vi "MathematicaHandlerBindTest.vi"() -> ()   [LabVIEW 2014]
uses:
  <vilib>/event_ctls.llb/lveventtype.ctl
panel:
  out "Array":string[](array[string])
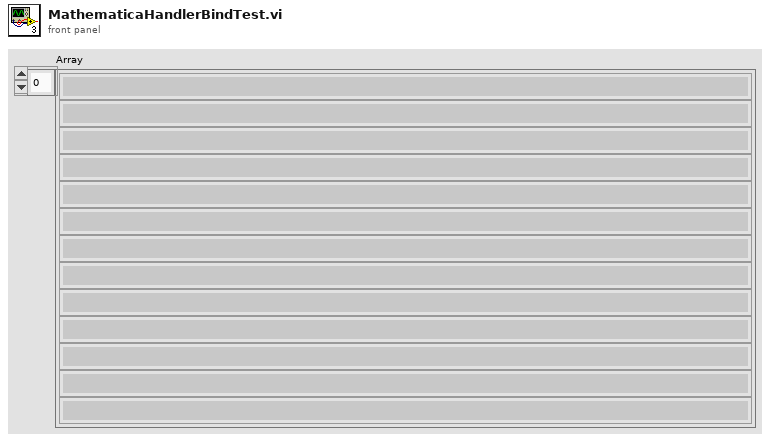
[diagram p1: front panel]
types:
  T1 = typedef "lveventtype.ctl" = enum32{"Null", "Timeout", "Annotation Menu Selection", "Annotation Menu Selection?", "App Instance Close", "App Instance Close?", "Autoscale Range Change", "Bookmark Info Change", "Cell Edit", "Cell Edit?", "Cursor Grab", "Cursor Grab?", "Cursor Menu Selection", "Cursor Menu Selection?", "Cursor Move", "Cursor Release", "Data Change", "Direction Change", "Display State Change", "Drag Ended", "Drag Enter", "Drag Leave", "Drag Over", "Drag Source Update", "Drag Starting", "Drag Starting?", "Drop", "Exec State Change", "Key Down", "Key Down?", "Key Repeat", "Key Repeat?", "Key Up", "Listbox Double Click", "Menu Activation?", "Menu Selection (App)", "Menu Selection? (App)", "Menu Selection (User)", "Mouse Down", "Mouse Down?", "Mouse Enter", "Mouse Leave", "Mouse Move", "Mouse Up", "Mouse Wheel", "NI Security User Change (App)", "Pane Size", "Panel Close", "Panel Close?", "Panel Resize", "Plot Attribute Change", "Scale Range Change", "Shortcut Menu Activation?", "Shortcut Menu Selection (App)", "Shortcut Menu Selection? (App)", "Shortcut Menu Selection (User)", "Tree Double Click", "Tree Drag", "Tree Drag?", "Tree Drop", "Tree Drop?", "Tree Item Close", "Tree Item Close?", "Tree Item Open", "Tree Item Open?", "User Event", "Value Change"}
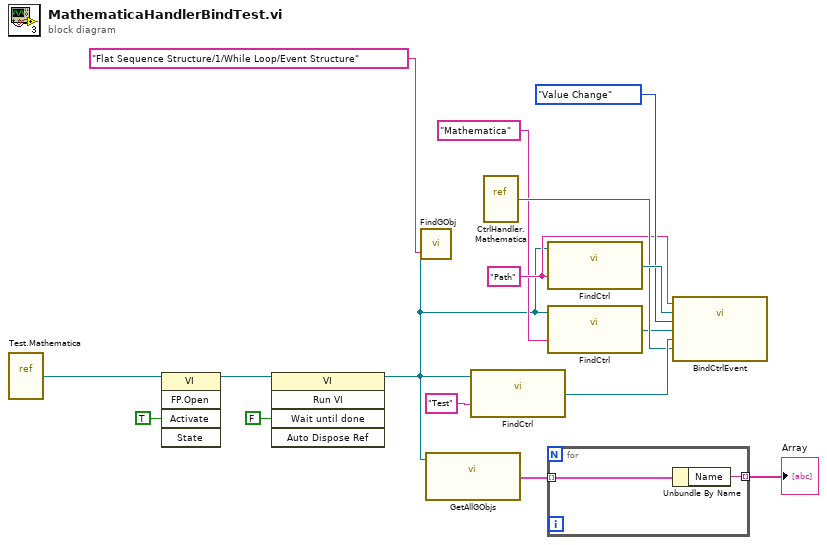
[diagram p0: block diagram]
diagram:
  w8 = "Path" ("Name")
  n1 = vi-ref "Test.Mathematica.vi"() -> (w6:refnum<vi>)
  n2 = invoke class="VI" method="FP.Open"(reference=w6, "Activate"=TRUE ("Activate?")) -> (reference out=w5:refnum<vi>)  [unwired: 3 in, 4 out]
  n3 = invoke class="VI" method="Run VI"(reference=w5, "Wait until done"=FALSE ("Wait Until Done")) -> (reference out=w2:refnum<vi>)  [unwired: 3 in, 4 out]
  n4 = call "FindGObj.vi"("Name"="Flat Sequence Structure/1/While Loop/Event Structure", "VI"=w2) -> ()  [unwired: 1 out]
  n5 = call "GetAllGObjs.vi"("VI"=w2) -> ("GObjs"=w16:cluster{"Name":string, "GObj":refnum<vi>}[])  [unwired: 1 in]
  n6 = call "FindCtrl.vi"("Name"="Test", "VI"=w2) -> ("Ctrl"=w10:refnum<vi>)
  n7 = vi-ref "CtrlHandler.Mathematica.vi"() -> (w9:refnum<vi>)
  n8 = call "FindCtrl.vi"("Name"=w8, "VI"=w2) -> ("Ctrl"=w13:refnum<vi>)
  n9 = call "FindCtrl.vi"("Name"="Mathematica", "VI"=w2) -> ("Ctrl"=w1:refnum<vi>)
  n10 = for {
    tunnel: w16 -> [w18] mode=indexing
    tunnel: [w17] -> w15 mode=indexing
    n11 = Unbundle By Name(w18) -> ("Name"=w17:string)
  }
  "Array" <- w15
  n12 = call "BindCtrlEvent.vi"("Stop"=w10, "VI"=w9, "Data"=w1, "Type"=lveventtype."Value Change", "Ctrl"=w13, "Name"=w8) -> ()  [unwired: 1 out]
